vi "emi_Or Error Bool.vi"(4 "error in":errorcluster, 5 "x":bool) -> (1 "x .or. Error?":bool)   [LabVIEW 2010]
doc: "ORs the boolm and the status of teh error cluster(Error = True)"
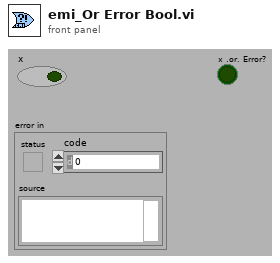
[diagram p1: front panel]
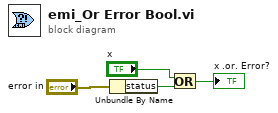
[diagram p0: block diagram]
diagram:
  n1 = Unbundle By Name("error in") -> ("status"=w2:bool)
  n2 = Or(x="x", y=w2) -> (x .or. y?=→"x .or. Error?":bool)
